vi "DATA_VI.vi"() -> ()   [LabVIEW 2022 SP3]
uses:
  TypeDefs/KoelOnOff.ctl
  TypeDefs/LogData.ctl
  <extravilib>/ChannelInstances/Tag-u16[MaskineON,MaskineSTOP,]/Write With Abort.vi
  <extravilib>/ChannelInstances/Tag-bool/Read With Abort.vi
  <extravilib>/ChannelInstances/Tag-dbl/Read With Abort.vi
  <extravilib>/ChannelInstances/Tag-t'KoelOnOff.ctl'/Write With Abort.vi
  <extravilib>/ChannelInstances/Tag-t'LogData.ctl'/Read With Abort.vi
  <extravilib>/ChannelInstances/Tag-u16[MaskineON,MaskineSTOP,]/Read With Abort.vi
  <extravilib>/ChannelInstances/Tag-t'KoelOnOff.ctl'/Read With Abort.vi
  <extravilib>/ChannelInstances/Tag-bool/Write With Abort.vi
  <extravilib>/ChannelInstances/Stream-t'LogData.ctl'/Read With Abort.vi
  <extravilib>/ChannelInstances/Tag-a[.](dbl)/Read With Abort.vi
  <extravilib>/ChannelInstances/Tag-dbl/Write With Abort.vi
  <extravilib>/ChannelInstances/Stream-a[.](dbl)/Read With Abort.vi
  <extravilib>/ChannelInstances/Stream-t'LogData.ctl'/Write With Abort.vi
  <extravilib>/ChannelInstances/Tag-t'LogData.ctl'/Write With Abort.vi
  <extravilib>/ChannelInstances/Stream-t'LogData.ctl'/EndpointRead.vi
  <extravilib>/ChannelInstances/Stream-a[.](dbl)/EndpointRead.vi
  <extravilib>/ChannelInstances/Stream-t'LogData.ctl'/Endpoint.vi
  <extravilib>/ChannelInstances/Stream-t'LogData.ctl'/Instantiate.vi
  <extravilib>/ChannelInstances/Stream-t'LogData.ctl'/)Channel.vi
  <resource>/ChannelSupport/_ChannelSupport/WaitIfNeeded.vi
  <extravilib>/ChannelInstances/Tag-dbl/Instantiate.vi
  <extravilib>/ChannelInstances/Tag-t'LogData.ctl'/Instantiate.vi
  <extravilib>/ChannelInstances/Tag-t'LogData.ctl'/EndpointRead.vi
  <extravilib>/ChannelInstances/Tag-t'KoelOnOff.ctl'/Instantiate.vi
  <extravilib>/ChannelInstances/Tag-dbl/EndpointRead.vi
  <extravilib>/ChannelInstances/Tag-t'KoelOnOff.ctl'/Endpoint.vi
  <extravilib>/ChannelInstances/Tag-bool/Instantiate.vi
  <extravilib>/ChannelInstances/Tag-bool/EndpointRead.vi
  <extravilib>/ChannelInstances/Tag-u16[MaskineON,MaskineSTOP,]/Instantiate.vi
  <extravilib>/ChannelInstances/Tag-u16[MaskineON,MaskineSTOP,]/EndpointRead.vi
  <extravilib>/ChannelInstances/Tag-t'KoelOnOff.ctl'/EndpointRead.vi
  <extravilib>/ChannelInstances/Tag-bool/Endpoint.vi
  <extravilib>/ChannelInstances/Tag-u16[MaskineON,MaskineSTOP,]/Endpoint.vi
  <extravilib>/ChannelInstances/Tag-a[.](dbl)/Instantiate.vi
  <extravilib>/ChannelInstances/Stream-a[.](dbl)/Instantiate.vi
  <extravilib>/ChannelInstances/Tag-a[.](dbl)/EndpointRead.vi
  <extravilib>/ChannelInstances/Tag-dbl/Endpoint.vi
  <extravilib>/ChannelInstances/Stream-a[.](dbl)/)Channel.vi
  <extravilib>/ChannelInstances/Tag-t'LogData.ctl'/Endpoint.vi
  <extravilib>/ChannelInstances/Stream-a[.](dbl).lvlib
  <extravilib>/ChannelInstances/Tag-dbl.lvlib
  <extravilib>/ChannelInstances/Tag-a[.](dbl).lvlib
  <extravilib>/ChannelInstances/Tag-u16[MaskineON,MaskineSTOP,].lvlib
  <extravilib>/ChannelInstances/Tag-bool.lvlib
  <extravilib>/ChannelInstances/Tag-t'KoelOnOff.ctl'.lvlib
  <extravilib>/ChannelInstances/Tag-t'LogData.ctl'.lvlib
  <extravilib>/ChannelInstances/Stream-t'LogData.ctl'.lvlib
panel:
  in  "stop 9":bool
  out "Tryk":T1(graph)
  out "Temp":T1(graph)
  out "element 3":enum16{"MaskineON", "MaskineSTOP", ""}(ring)
  out "element 2":T2
  in  "stop 8":bool
  in  "Gem og log data":bool
  out "Waveform Chart":dbl(graph)
  out "u":dbl
  in  "Set punkt":dbl
  in  "Fejl on":dbl
  in  "k_d":dbl
  in  "k_i":dbl
  in  "k_p":dbl
  in  "stop 7":bool
  out "Ventil":bool
  out "Kompressor":bool
  in  "stop 6":bool
  in  "stop 5":bool
  in  "stop 3":bool
  in  "Motor":bool
  in  "Pumpe":bool
  in  "Maskine Stop":bool
  in  "Maskine ON":bool
  out "Termister":dbl[](array[numeric])
  out "Tryk_Hoej":dbl[](array[numeric])
  out "Tryk_Lav":dbl[](array[numeric])
  out "element":dbl
  in  "stop 2":bool
  in  "stop":bool
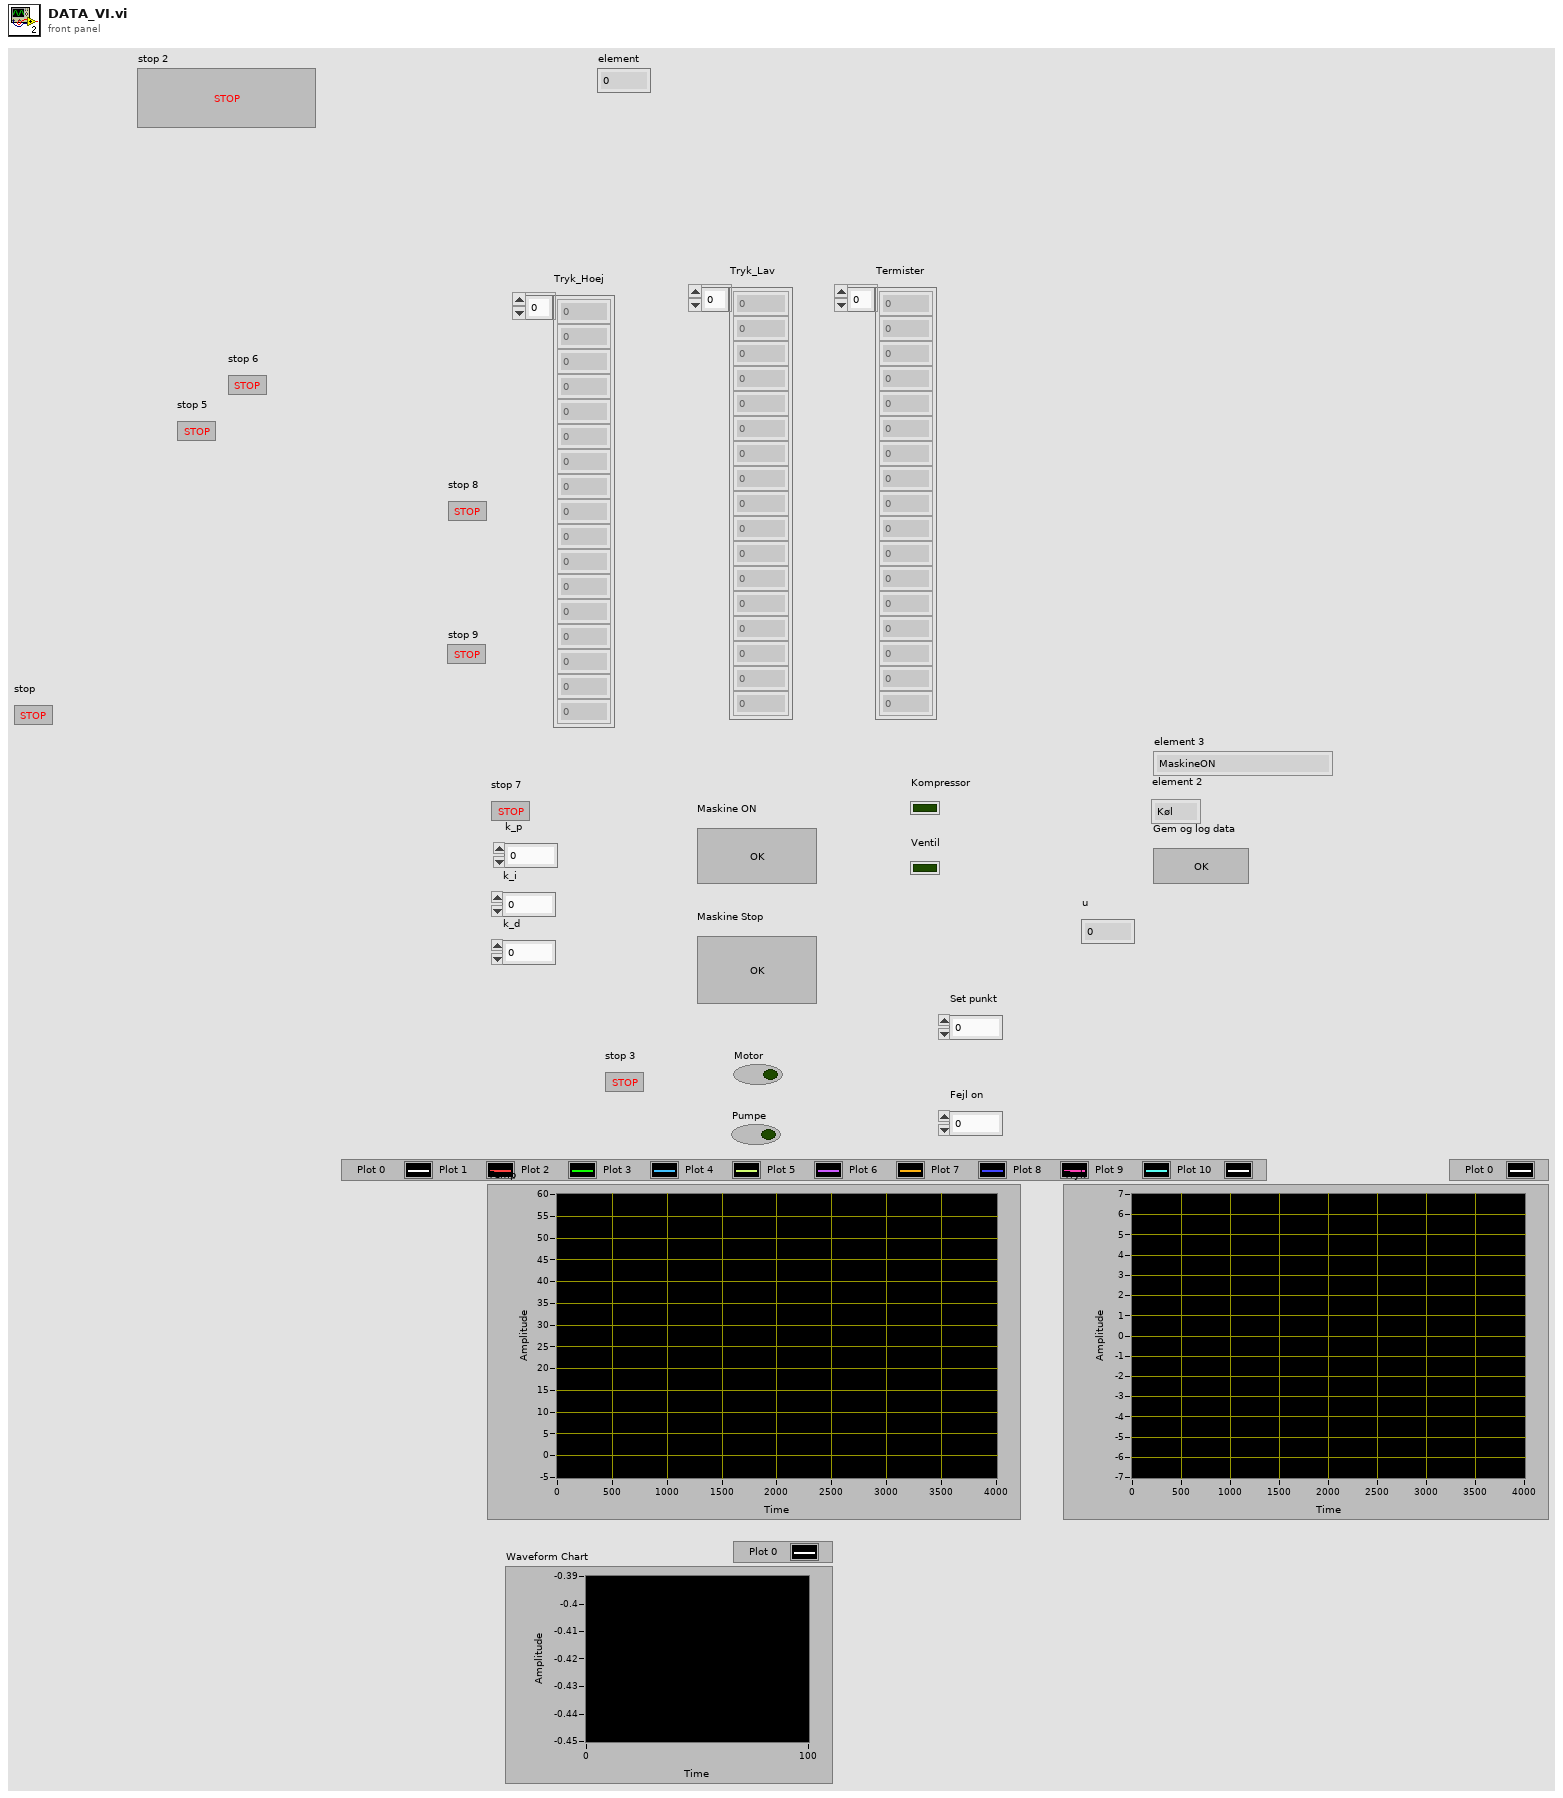
[diagram p1: front panel]
types:
  T1 = cluster{"TID ARRAY (X)":dbl[], "Termister_rum":dbl[]}[]
  T2 = typedef "KoelOnOff.ctl" = enum16{"Køl", "IkkeKøl"}
  T3 = typedef "Tag-a[.](dbl).lvlib/))Channel.ctl" = refnum<queue>
  T4 = typedef "Tag-dbl.lvlib/))Channel.ctl" = refnum<queue>
  T5 = typedef "Stream-a[.](dbl).lvlib/)Channel.ctl" = refnum<queue>
  T6 = typedef "LogData.ctl" = cluster{"DAQ1":cluster{"Brine":dbl[], "Kondensator_LUFT":dbl[], "Motor":dbl[], "TID ARRAY (X)":dbl[]}, "DAQ2":cluster{"Efter_EVAP":dbl[], "Kompressor":dbl[], "Efter Expansion":dbl[], "TID ARRAY (X)":dbl[]}, "DAQ3":cluster{"Slush":dbl[], "E-KOMP":dbl[], "Efter_kond":dbl[], "TID ARRAY (X)":dbl[]}, "Termister_rum":dbl[], "Tryk_Lav2":dbl[], "Tryk_hoej":dbl[]}
  T7 = cluster{"Slush":dbl[], "E-KOMP":dbl[], "Efter_kond":dbl[], "TID ARRAY (X)":dbl[]}
  T8 = cluster{"Efter_EVAP":dbl[], "Kompressor":dbl[], "Efter Expansion":dbl[], "TID ARRAY (X)":dbl[]}
  T9 = cluster{"Brine":dbl[], "Kondensator_LUFT":dbl[], "Motor":dbl[], "TID ARRAY (X)":dbl[]}
  T10 = typedef "Tag-t'LogData.ctl'.lvlib/))Channel.ctl" = refnum<queue>
  T11 = typedef "Stream-t'LogData.ctl'.lvlib/)Channel.ctl" = refnum<queue>
  T12 = typedef "Tag-bool.lvlib/))Channel.ctl" = refnum<queue>
  T13 = typedef "Tag-u16[MaskineON,MaskineSTOP,].lvlib/))Channel.ctl" = refnum<queue>
  T14 = enum16{"I_REG", "ID_REG", "P_REG", "PI_REG", "PD_REG", "PID_REG"}
  T15 = typedef "Tag-t'KoelOnOff.ctl'.lvlib/))Channel.ctl" = refnum<queue>
  T16 = cluster{"TID ARRAY (X)":dbl[], "Tryk_hoej":dbl[]}
  T17 = cluster{"TID ARRAY (X)":dbl[], "Kondensator_LUFT":dbl[]}
  T18 = cluster{"TID ARRAY (X)":dbl[], "Efter_EVAP":dbl[]}
  T19 = cluster{"TID ARRAY (X)":dbl[], "Kompressor":dbl[]}
  T20 = cluster{"TID ARRAY (X)":dbl[], "Efter Expansion":dbl[]}
  T21 = cluster{"TID ARRAY (X)":dbl[], "Efter_kond":dbl[]}
  T22 = cluster{"TID ARRAY (X)":dbl[], "Termister_rum":dbl[]}
  T23 = cluster{"TID ARRAY (X)":dbl[], "Tryk_Lav2":dbl[]}
  T24 = cluster{"TID ARRAY (X)":dbl[], "Tryk_hoej":dbl[]}[]
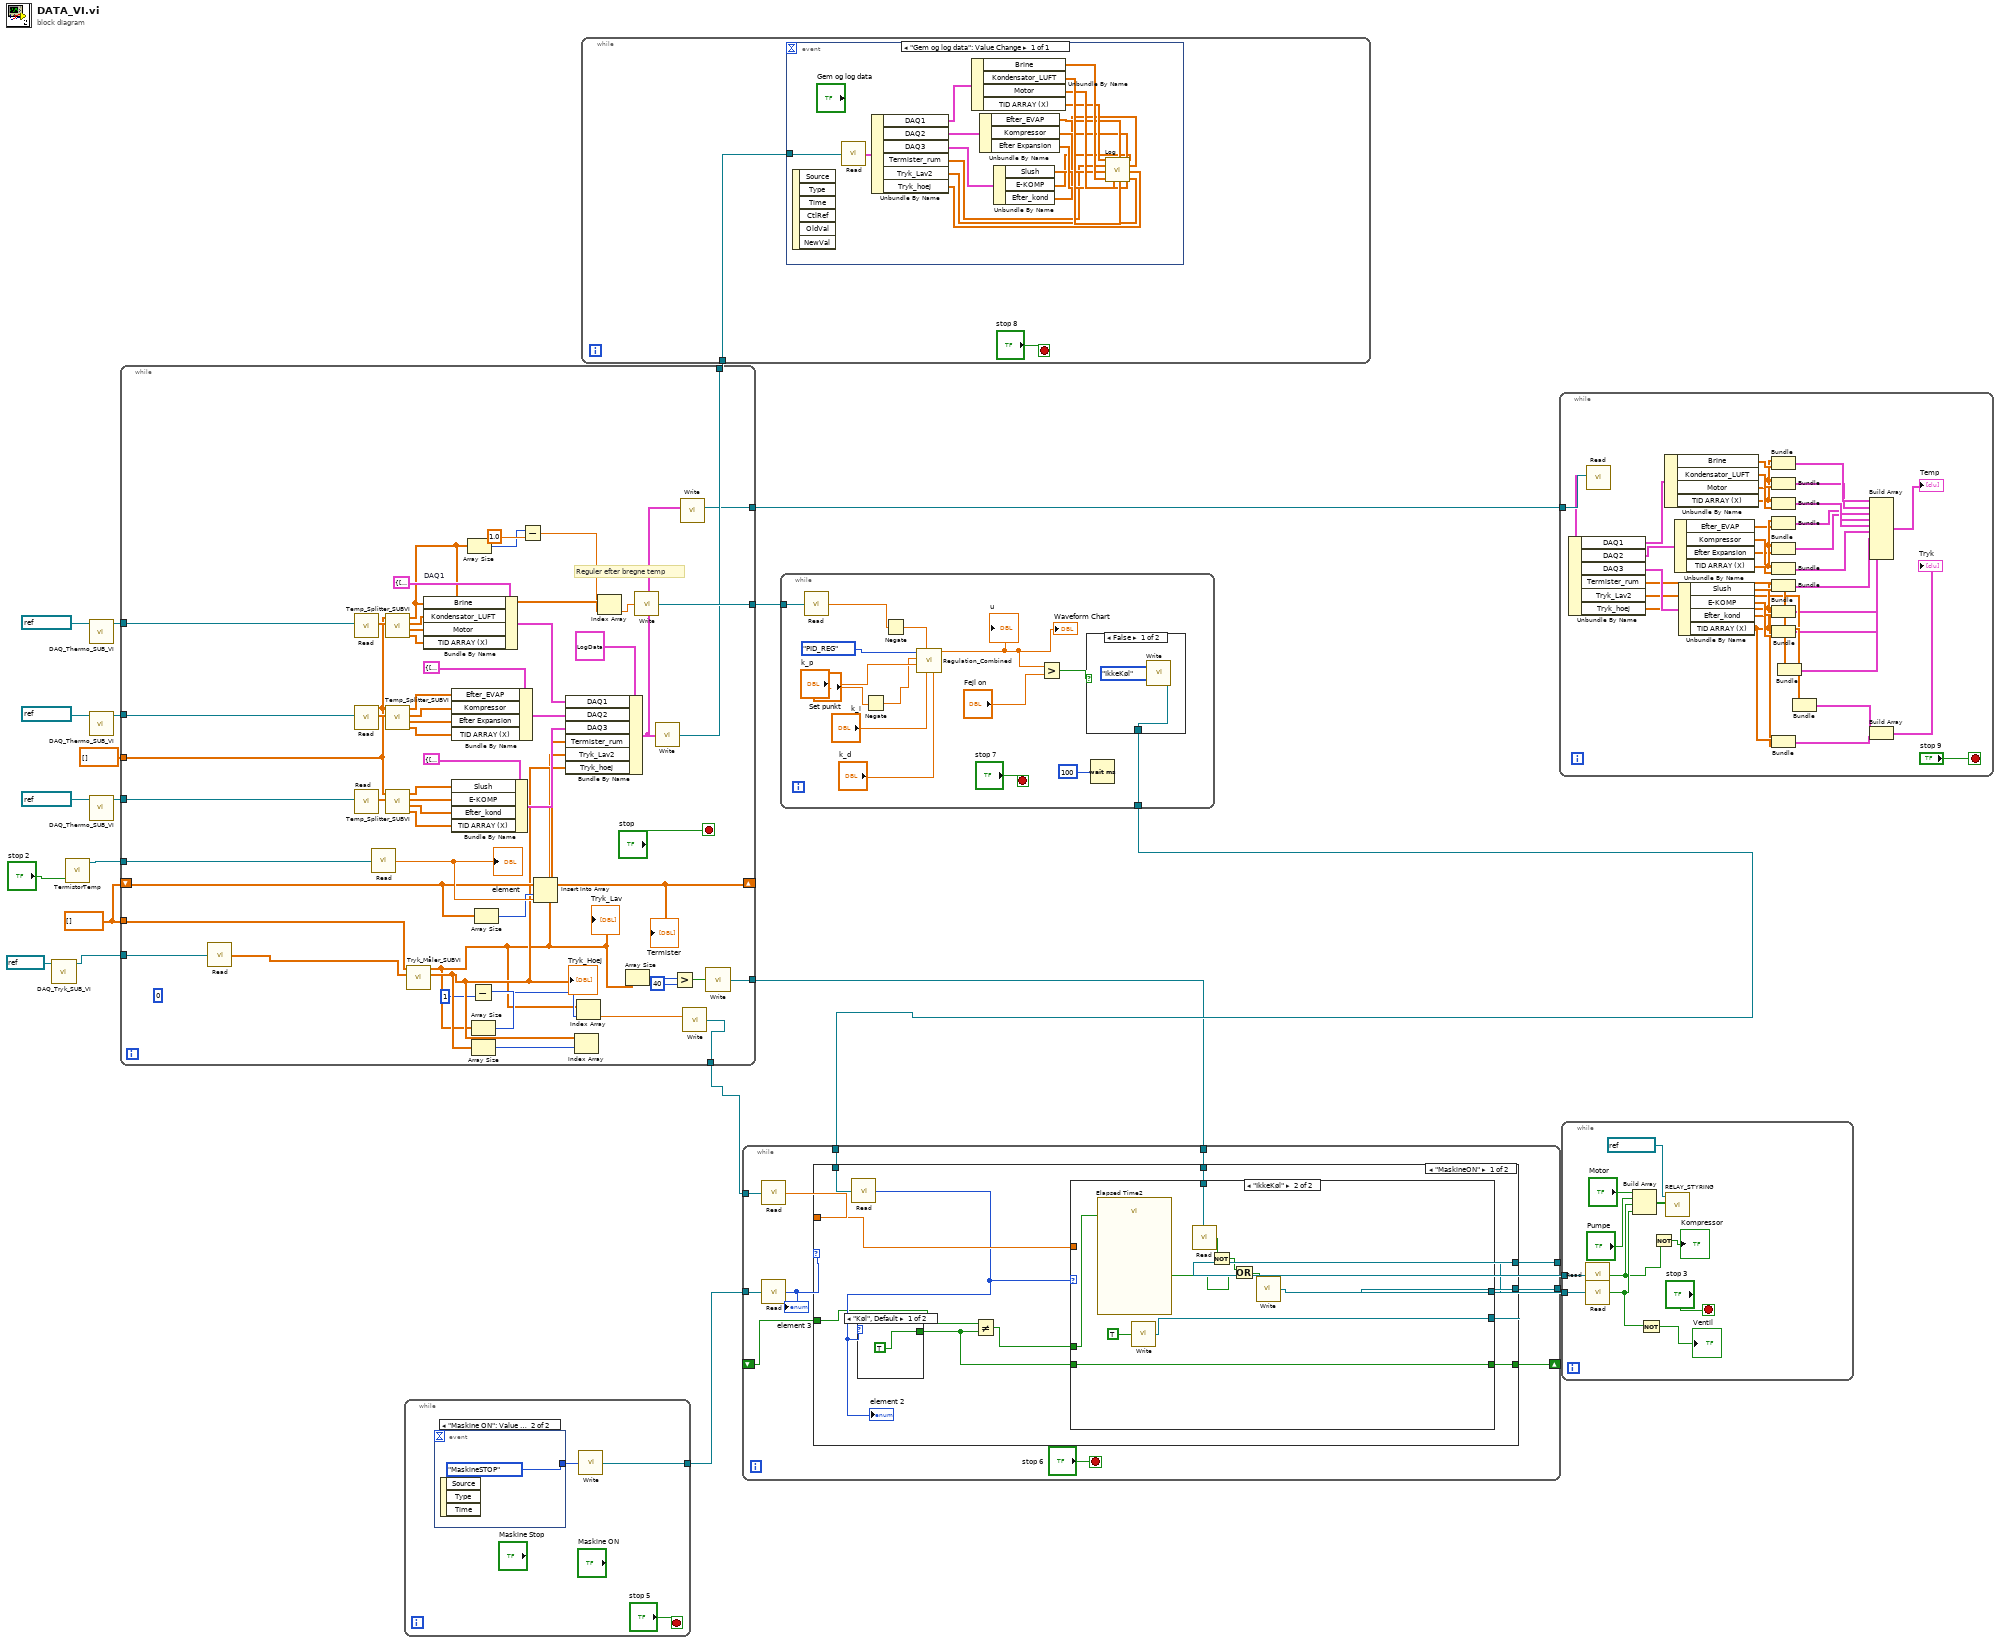
[diagram p0: block diagram]
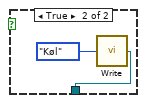
[diagram p2: hidden frame]
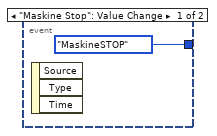
[diagram p3: hidden frame]
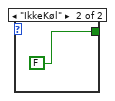
[diagram p4: hidden frame]
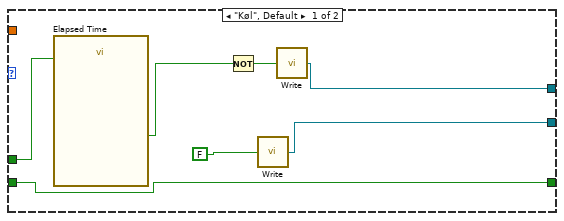
[diagram p5: hidden frame]
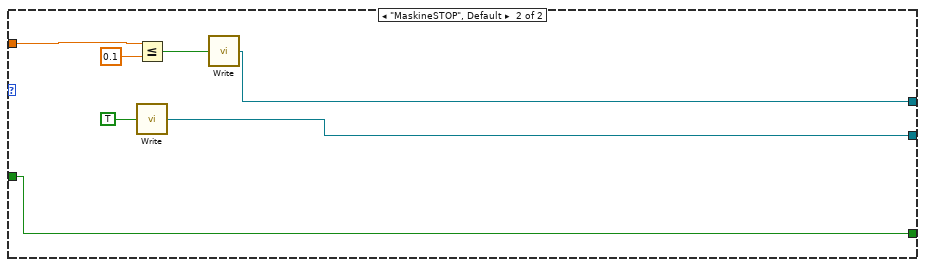
[diagram p6: hidden frame]
diagram:
  w10 = dbl[] []
  n1 = call "DAQ_Tryk_SUB_VI.vi"("task in"=refnum<k21> "Tryk") -> ("channel"=w11:T3)  [unwired: 10 in]
  n2 = call "TermistorTemp.vi"("stop"="stop 2") -> ("channel"=w13:T4)  [unwired: 3 in, 1 out]
  n3 = call "DAQ_Thermo_SUB_VI.vi"("task in"=refnum<k21> "DAQ_1") -> ("channel"=w18:T5)  [unwired: 10 in]
  n4 = call "DAQ_Thermo_SUB_VI.vi"("task in"=refnum<k21> "DAQ_2") -> ("channel"=w16:T5)  [unwired: 10 in]
  n5 = call "DAQ_Thermo_SUB_VI.vi"("task in"=refnum<k21> "DAQ_3") -> ("channel"=w17:T5)  [unwired: 10 in]
  n6 = while {
    tunnel: w18 -> [w75]
    tunnel: w17 -> [w73]
    tunnel: w16 -> [w72]
    tunnel: dbl[] [] -> [w69]
    tunnel: w13 -> [w50]
    tunnel: w10 -> [w47]
    tunnel: w11 -> [w49]
    shift-right: [w39] -> _
    shift-left: w10 -> [w45]
    tunnel: [w40] -> w6
    tunnel: [w36] -> w4
    tunnel: [w35] -> w3
    tunnel: [w33] -> w2
    tunnel: [w22] -> w1
    stop <- "stop" stop-if-true
    (unwired) 0 ("index")
    # "Reguler efter bregne temp"
    n7 = call <extravilib>:"Read.vi"("channel"=w49) -> ("element"=w48:dbl[])  [unwired: 1 in, 1 out]
    n8 = call <extravilib>:"Read.vi"("channel"=w75) -> ("element"=w74:dbl[])  [unwired: 6 in, 4 out]
    n9 = call <extravilib>:"Read.vi"("channel"=w72) -> ("element"=w70:dbl[])  [unwired: 6 in, 4 out]
    n10 = call <extravilib>:"Read.vi"("channel"=w73) -> ("element"=w71:dbl[])  [unwired: 6 in, 4 out]
    n11 = call <extravilib>:"Read.vi"("channel"=w50) -> ("element"=w46:dbl)  [unwired: 1 in, 1 out]
    "element" <- w46
    n12 = call "Temp_Splitter_SUBVI.vi"("DAQ_OUT"=w74, "Tomt Array"=w69) -> ("Counter_Array"=w65:dbl[], "TEMP3"=w66:dbl[], "TEMP2"=w67:dbl[], "TEMP1"=w42:dbl[])  [unwired: 6 in]
    n13 = call "Temp_Splitter_SUBVI.vi"("DAQ_OUT"=w70, "Tomt Array"=w69) -> ("Counter_Array"=w60:dbl[], "TEMP3"=w61:dbl[], "TEMP2"=w62:dbl[], "TEMP1"=w63:dbl[])  [unwired: 6 in]
    n14 = call "Temp_Splitter_SUBVI.vi"("DAQ_OUT"=w71, "Tomt Array"=w69) -> ("Counter_Array"=w55:dbl[], "TEMP3"=w56:dbl[], "TEMP2"=w57:dbl[], "TEMP1"=w58:dbl[])  [unwired: 6 in]
    n15 = call "Tryk_Måler_SUBVI.vi"("element"=w48, "Array in"=w47) -> ("Tryk_Hoej"=w38:dbl[], "Tryk_Lav"=w26:dbl[])  [unwired: 8 in]
    "Tryk_Lav" <- w26
    "Tryk_Hoej" <- w38
    n16 = Bundle By Name "DAQ1"(cluster=T9 {"Brine"=[], "Kondensator_LUFT"=[], "Motor"=[], "TID ARRAY (X)"=[]} ("input cluster"), "Brine"=w42, "Kondensator_LUFT"=w67, "Motor"=w66, "TID ARRAY (X)"=w65) -> (w54:T9)
    n17 = Bundle By Name(cluster=T8 {"Efter_EVAP"=[], "Kompressor"=[], "Efter Expansion"=[], "TID ARRAY (X)"=[]} ("input cluster"), "Efter_EVAP"=w63, "Kompressor"=w62, "Efter Expansion"=w61, "TID ARRAY (X)"=w60) -> (w53:T8)
    n18 = Bundle By Name(cluster=T7 {"Slush"=[], "E-KOMP"=[], "Efter_kond"=[], "TID ARRAY (X)"=[]} ("input cluster"), "Slush"=w58, "E-KOMP"=w57, "Efter_kond"=w56, "TID ARRAY (X)"=w55) -> (w52:T7)
    n19 = Array Size(array=w42) -> (size(s)=w31:i32)
    n20 = Array Size(array=w26) -> (size(s)=w29:i32)
    n21 = Subtract(x=w29, y=1) -> (x-y=w27:i32)
    n22 = Array Size(array=w38) -> (size(s)=w43:i32)
    n23 = Array Size(array=w45) -> (size(s)=w44:i32)
    n24 = Subtract(x=w31, y=1.0) -> (x-y=w30:dbl)
    n25 = Insert Into Array(array=w45, index=w44, new element=w46) -> (w39:dbl[])
    "Termister" <- w39
    n26 = Bundle By Name(cluster=T6 {"DAQ1"={"Brine"=[], "Kondensator_LUFT"=[], "Motor"=[], "TID ARRAY (X)"=[]}, "DAQ2"={"Efter_EVAP"=[], "Kompressor"=[], "Efter Expansion"=[], "TID ARRAY (X)"=[]}, "DAQ3"={"Slush"=[], "E-KOMP"=[], "Efter_kond"=[], "TID ARRAY (X)"=[]}, "Termister_rum"=[], "Tryk_Lav2"=[], "Tryk_hoej"=[]} ("input cluster"), "DAQ1"=w54, "DAQ2"=w53, "DAQ3"=w52, "Termister_rum"=w39, "Tryk_Lav2"=w26, "Tryk_hoej"=w38) -> (w37:T6)
    n27 = Index Array(array=w38, index=w43) -> ()  [unwired: 1 out]
    n28 = Index Array(array=w26, index=w27) -> (element=w34:dbl)
    n29 = Index Array(array=w42, index=w30) -> (element=w41:dbl)
    n30 = Array Size(array=w26) -> (size(s)=w25:i32)
    n31 = call <extravilib>:"Write.vi"("element"=w41) -> ("channel"=w40:T4)  [unwired: 1 out]
    n32 = call <extravilib>:"Write.vi"("element"=w37) -> ("channel"=w36:T10)  [unwired: 1 out]
    n33 = Greater?(x=w25, y=40) -> (0:w23:bool)
    n34 = call <extravilib>:"Write.vi"("element"=w37) -> ("channel"=w33:T11)  [unwired: 8 in, 2 out]
    n35 = call <extravilib>:"Write.vi"("element"=w34) -> ("channel"=w35:T4)  [unwired: 1 out]
    n36 = call <extravilib>:"Write.vi"("element"=w23) -> ("channel"=w22:T12)  [unwired: 1 out]
  }
  n37 = while {
    tunnel: [w78] -> w9
    stop <- "stop 5" stop-if-true
    n38 = event shown="[1] \"Maskine ON\": Value Change" {
      selector: _ -> [_ _]
      dyn-events: _ -> [_ _]
      timeout: _ -> [_ _]
      tunnel: [enum16{"MaskineON", "MaskineSTOP", ""}."MaskineSTOP" enum16{"MaskineON", "MaskineSTOP"}."MaskineSTOP"] -> w79
      event "Maskine Stop": Value Change {
        n39 = event-data() -> ()  [unwired: 1 in, 3 out]
      }
      event "Maskine ON": Value Change {
        n40 = event-data() -> ()  [unwired: 1 in, 3 out]
      }
    }
    n41 = call <extravilib>:"Write.vi"("element"=w79) -> ("channel"=w78:T13)  [unwired: 1 out]
  }
  n42 = while {
    tunnel: w4 -> [w83]
    stop <- "stop 8" stop-if-true
    n43 = event shown="[0] \"Gem og log data\": Value Change" {
      selector: _ -> [_]
      dyn-events: _ -> [_]
      timeout: _ -> [_]
      tunnel: w83 -> [w88]
      event "Gem og log data": Value Change {
        n44 = event-data() -> ()  [unwired: 1 in, 6 out]
        n45 = call <extravilib>:"Read.vi"("channel"=w88) -> ("element"=w87:T6)  [unwired: 1 in, 1 out]
        n46 = Unbundle By Name(w87) -> ("DAQ1"=w101:T9, "DAQ2"=w96:T8, "DAQ3"=w95:T7, "Termister_rum"=w86:dbl[], "Tryk_Lav2"=w85:dbl[], "Tryk_hoej"=w84:dbl[])
        n47 = Unbundle By Name(w101) -> ("Brine"=w100:dbl[], "Kondensator_LUFT"=w99:dbl[], "Motor"=w98:dbl[], "TID ARRAY (X)"=w97:dbl[])
        n48 = Unbundle By Name(w96) -> ("Efter_EVAP"=w94:dbl[], "Kompressor"=w93:dbl[], "Efter Expansion"=w92:dbl[])
        n49 = Unbundle By Name(w95) -> ("Slush"=w91:dbl[], "E-KOMP"=w89:dbl[], "Efter_kond"=w90:dbl[])
        n50 = call "Log.vi"("Iterationer"=w97, "Rumtemperatur"=w86, "Slush Ice"=w91, "Brine"=w100, "Motor"=w98, "Efter ForD"=w94, "Kond luft"=w99, "Komp"=w93, "Efter EPV"=w92, "Efter Komp"=w89, "Efter Kond"=w90, "Tryk hoej"=w84, "Tryk lav"=w85) -> ()  [unwired: 15 in]
      }
    }
  }
  n51 = while {
    tunnel: w6 -> [w115]
    tunnel: [w108] -> w5
    stop <- "stop 7" stop-if-true
    n52 = call <extravilib>:"Read.vi"("channel"=w115) -> ("element"=w102:dbl)  [unwired: 1 in, 1 out]
    n53 = Negate(x="Set punkt") -> (-x=w103:dbl)
    n54 = Negate(x=w102) -> (-x=w105:dbl)
    n55 = call "Regulation_Combined.vi"("k_d"="k_d", "k_i"="k_i", "DATA"=w105, "k_p"="k_p", "SP"=w103, "Regulation type"=T14."PID_REG") -> ("u"=w107:dbl)  [unwired: 2 in, 3 out]
    "u" <- w107
    "Waveform Chart" <- w107
    n56 = Greater?(x=w107, y="Fejl on") -> (0:w109:bool)
    n57 = case shown="False" w109 {
      tunnel: [w117 w119] -> w108
      frame False {
        n58 = call <extravilib>:"Write.vi"("element"=KoelOnOff."IkkeKøl") -> ("channel"=w117:T15)  [unwired: 1 out]
      }
      frame True {
        n59 = call <extravilib>:"Write.vi"("element"=KoelOnOff."Køl") -> ("channel"=w119:T15)  [unwired: 1 out]
      }
    }
    n60 = Wait (ms)(milliseconds to wait=u32 100) -> ()  [unwired: 1 out]
  }
  n61 = while {
    tunnel: w3 -> [w131]
    tunnel: w9 -> [w130]
    tunnel: [w127] -> w8
    tunnel: [w126] -> w7
    tunnel: w5 -> [w124]
    shift-right: [w123] -> _
    shift-left: _ -> [w122]
    tunnel: w1 -> [w121]
    stop <- "stop 6" stop-if-true
    n62 = call <extravilib>:"Read.vi"("channel"=w131) -> ("element"=w128:dbl)  [unwired: 1 in, 1 out]
    n63 = call <extravilib>:"Read.vi"("channel"=w130) -> ("element"=w129:enum16{"MaskineON", "MaskineSTOP", ""})  [unwired: 1 in, 1 out]
    "element 3" <- w129
    n64 = case shown="\"MaskineON\"" w129 {
      tunnel: w128 -> [w141 w163]
      tunnel: [w140 w164] -> w127
      tunnel: [w139 w162] -> w126
      tunnel: w124 -> [w138 _]
      tunnel: [w136 w161] -> w123
      tunnel: w122 -> [w135 w161]
      tunnel: w121 -> [w132 _]
      frame "MaskineON" {
        n65 = call <extravilib>:"Read.vi"("channel"=w138) -> ("element"=w137:T2)  [unwired: 1 in, 1 out]
        "element 2" <- w137
        n66 = case shown="\"Køl\", Default" w137 {
          tunnel: [TRUE FALSE] -> w134
          frame "Køl", Default {
          }
          frame "IkkeKøl" {
          }
        }
        n67 = Not Equal?(x=w135, y=w134) -> (x != y?=w133:bool)
        n68 = case shown="\"IkkeKøl\"" w137 {
          tunnel: w141 -> [_ _]
          tunnel: [w150 w159] -> w140
          tunnel: [w149 w160] -> w139
          tunnel: w134 -> [w144 w157]
          tunnel: [w144 w157] -> w136
          tunnel: w133 -> [w147 w156]
          tunnel: w132 -> [_ w155]
          frame "Køl", Default {
            n69 = call "Elapsed Time"("Reset"=w147) -> ("Time has Elapsed"=w146:bool)  [unwired: 11 in, 7 out]
            n70 = Not(x=w146) -> (.not. x?=w145:bool)
            n71 = call <extravilib>:"Write.vi"("element"=FALSE) -> ("channel"=w150:T12)  [unwired: 1 out]
            n72 = call <extravilib>:"Write.vi"("element"=w145) -> ("channel"=w149:T12)  [unwired: 1 out]
          }
          frame "IkkeKøl" {
            n73 = call "Elapsed Time2"("Reset"=w156) -> ("Time has Elapsed"=w152:bool)  [unwired: 11 in, 7 out]
            n74 = call <extravilib>:"Write.vi"("element"=TRUE) -> ("channel"=w159:T12)  [unwired: 1 out]
            n75 = call <extravilib>:"Read.vi"("channel"=w155) -> ("element"=w154:bool)  [unwired: 1 in, 1 out]
            n76 = Not(x=w154) -> (.not. x?=w153:bool)
            n77 = Or(x=w153, y=w152) -> (x .or. y?=w151:bool)
            n78 = call <extravilib>:"Write.vi"("element"=w151) -> ("channel"=w160:T12)  [unwired: 1 out]
          }
        }
      }
      frame "MaskineSTOP", Default {
        n79 = Less Or Equal?(x=w163, y=0.1) -> (x <= y?=w165:bool)
        n80 = call <extravilib>:"Write.vi"("element"=TRUE) -> ("channel"=w164:T12)  [unwired: 1 out]
        n81 = call <extravilib>:"Write.vi"("element"=w165) -> ("channel"=w162:T12)  [unwired: 1 out]
      }
    }
  }
  n82 = while {
    tunnel: w2 -> [w202]
    stop <- "stop 9" stop-if-true
    n83 = call <extravilib>:"Read.vi"("channel"=w202) -> ("element"=w201:T6)  [unwired: 6 in, 4 out]
    n84 = Unbundle By Name(w201) -> ("DAQ1"=w200:T9, "DAQ2"=w195:T8, "DAQ3"=w190:T7, "Termister_rum"=w186:dbl[], "Tryk_Lav2"=w184:dbl[], "Tryk_hoej"=w183:dbl[])
    n85 = Unbundle By Name(w200) -> ("Brine"=w199:dbl[], "Kondensator_LUFT"=w198:dbl[], "Motor"=w197:dbl[], "TID ARRAY (X)"=w196:dbl[])
    n86 = Unbundle By Name(w195) -> ("Efter_EVAP"=w193:dbl[], "Kompressor"=w192:dbl[], "Efter Expansion"=w191:dbl[], "TID ARRAY (X)"=w194:dbl[])
    n87 = Unbundle By Name(w190) -> ("Slush"=w189:dbl[], "E-KOMP"=w188:dbl[], "Efter_kond"=w187:dbl[], "TID ARRAY (X)"=w185:dbl[])
    n88 = Bundle("TID ARRAY (X)"=w185, "Tryk_hoej"=w183) -> (w181:T16)  [unwired: 1 in]
    n89 = Bundle("TID ARRAY (X)"=w196, "Brine"=w199) -> (w180:cluster{"TID ARRAY (X)":dbl[], "Brine":dbl[]})  [unwired: 1 in]
    n90 = Bundle("TID ARRAY (X)"=w196, "Kondensator_LUFT"=w198) -> (w179:T17)  [unwired: 1 in]
    n91 = Bundle("TID ARRAY (X)"=w196, "Motor"=w197) -> (w178:cluster{"TID ARRAY (X)":dbl[], "Motor":dbl[]})  [unwired: 1 in]
    n92 = Bundle("TID ARRAY (X)"=w194, "Efter_EVAP"=w193) -> (w177:T18)  [unwired: 1 in]
    n93 = Bundle("TID ARRAY (X)"=w194, "Kompressor"=w192) -> (w176:T19)  [unwired: 1 in]
    n94 = Bundle("TID ARRAY (X)"=w194, "Efter Expansion"=w191) -> (w175:T20)  [unwired: 1 in]
    n95 = Bundle("TID ARRAY (X)"=w185, "Slush"=w189) -> (w174:cluster{"TID ARRAY (X)":dbl[], "Slush":dbl[]})  [unwired: 1 in]
    n96 = Bundle("TID ARRAY (X)"=w185, "E-KOMP"=w188) -> (w173:cluster{"TID ARRAY (X)":dbl[], "E-KOMP":dbl[]})  [unwired: 1 in]
    n97 = Bundle("TID ARRAY (X)"=w185, "Efter_kond"=w187) -> (w172:T21)  [unwired: 1 in]
    n98 = Bundle("TID ARRAY (X)"=w185, "Termister_rum"=w186) -> (w171:T22)  [unwired: 1 in]
    n99 = Bundle("TID ARRAY (X)"=w185, "Tryk_Lav2"=w184) -> (w182:T23)  [unwired: 1 in]
    n100 = Build Array(w180, w179, w178, w177, w176, w175, w174, w173, w172, w171) -> (→"Temp":T1)
    n101 = Build Array(w182, w181) -> (→"Tryk":T24)
  }
  n102 = while {
    tunnel: w8 -> [w208]
    tunnel: w7 -> [w207]
    stop <- "stop 3" stop-if-true
    n103 = call <extravilib>:"Read.vi"("channel"=w207) -> ("element"=w204:bool)  [unwired: 1 in, 1 out]
    n104 = call <extravilib>:"Read.vi"("channel"=w208) -> ("element"=w206:bool)  [unwired: 1 in, 1 out]
    n105 = Build Array("Motor", "Pumpe", w204, w206) -> (w210:bool[])
    n106 = Not(x=w206) -> (.not. x?=→"Ventil":bool)
    n107 = Not(x=w204) -> (.not. x?=→"Kompressor":bool)
    n108 = call "RELAY_STYRING.vi"("data"=w210, "task/channels in"=refnum<k21> "RELAY") -> ()  [unwired: 10 in]
  }
